vi "Swerve Autonomous.vi"(4 "Alternate Stop":bool, 6 "Robot Centric?":bool, 7 "Duration (sec)":dbl, 8 "Error In":errorcluster, 9 "Z":dbl, 10 "Y":dbl, 11 "X":dbl) -> (0 "Error Out":errorcluster)   [LabVIEW 2017]
panel:
  # "Swerve Autonomous\nFRC Team 34"
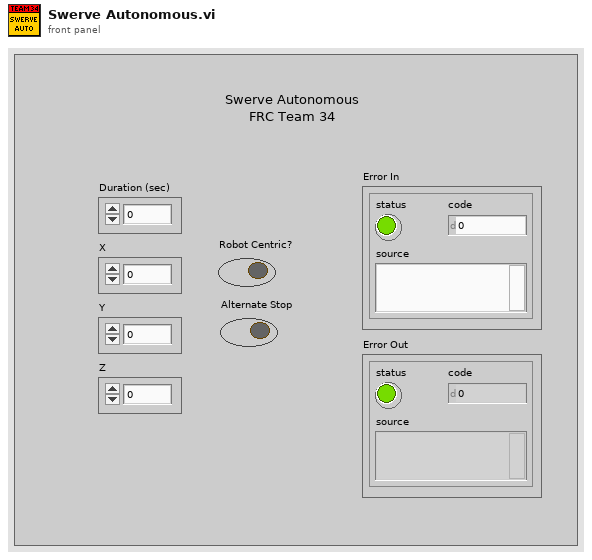
[diagram p1: front panel]
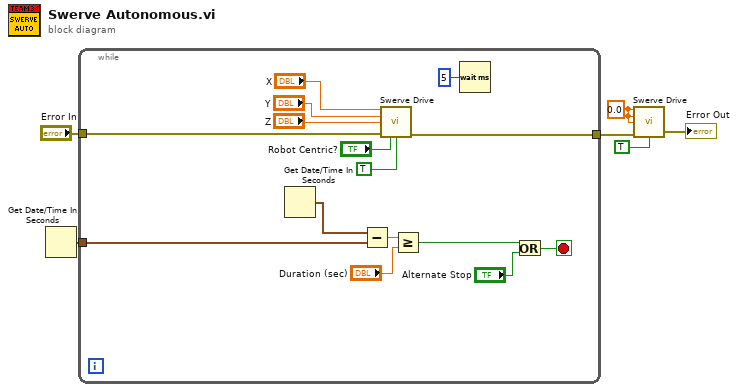
[diagram p0: block diagram]
diagram:
  w3 = 0.0 ("X")
  n1 = Get Date/Time In Seconds() -> (seconds since 1Jan1904=w6:timestamp)
  n2 = while {
    tunnel: w6 -> [w20]
    tunnel: "Error In" -> [w11]
    tunnel: [w10] -> w4
    stop <- w21 stop-if-true
    n3 = Get Date/Time In Seconds() -> (seconds since 1Jan1904=w19:timestamp)
    n4 = Subtract(x=w19, y=w20) -> (x-y=w18:dbl)
    n5 = call "Swerve Drive.vi"("X"="X", "Y"="Y", "Z"="Z", "Error In"=w11, "Robot Centric?"="Robot Centric?", "Autonomous?"=TRUE) -> ("Error Out"=w10:errorcluster)  [unwired: 5 in, 4 out]
    n6 = Greater Or Equal?(x=w18, y="Duration (sec)") -> (x >= y?=w7:bool)
    n7 = Wait (ms)(milliseconds to wait=u32 5) -> ()  [unwired: 1 out]
    n8 = Or(x=w7, y="Alternate Stop") -> (x .or. y?=w21:bool)
  }
  n9 = call "Swerve Drive.vi"("X"=w3, "Y"=w3, "Z"=w3, "Error In"=w4, "Autonomous?"=TRUE) -> ("Error Out"=→"Error Out":errorcluster)  [unwired: 6 in, 4 out]
